vi "Close Session.vi"(8 "error in":errorcluster, 10 "Session In":T1, 11 "Text Session":refnum<class "Text Device Session.lvclass">) -> (0 "error out":errorcluster, 2 "Session Out":T1)   [LabVIEW 2018, in "Text Device Session.lvclass"]
uses:
  Text Device Session.lvclass
  <vilib>/MSR Consulting, LLC/General Reuse/Session APIs/_Session Fwk/Typedefs/Session Handle.ctl
  <vilib>/MSR Consulting, LLC/General Reuse/Session APIs/_Session Fwk/Session - Root.lvclass
  C:/Program Files (x86)/National Instruments/LabVIEW 2018/vi.lib/MSR Consulting, LLC/General Reuse/Session APIs/_Session Fwk/Session - Root.lvclass
  File Access/Config Data/Config Data.lvclass
  Session Log/System Log.lvclass
  Text Device Session.lvclass/Text Device Session.ctl
  Read hSysLog.vi
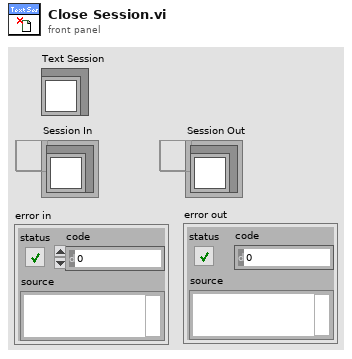
[diagram p1: front panel]
types:
  T1 = typedef "Session - Root.lvclass/Session Handle.ctl" = refnum<data-value>
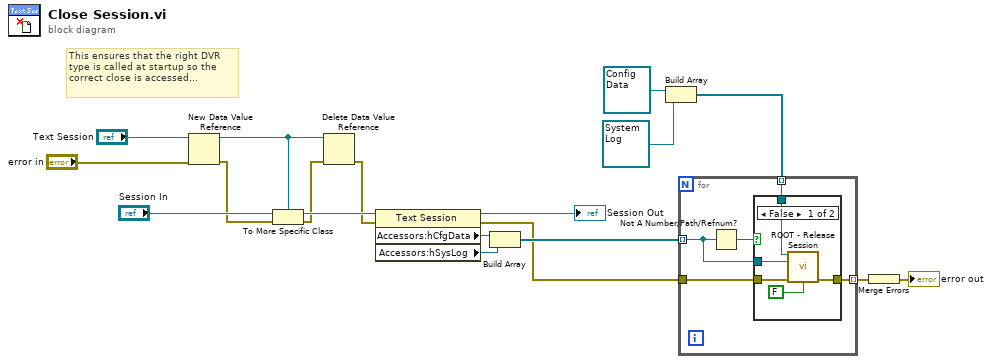
[diagram p0: block diagram]
diagram:
  # "This ensures that the right DVR type is called at startup so the correct close is accessed..."
  n1 = New Data Value Reference(data value="Text Session", error in="error in") -> (data value reference=w6:refnum<data-value>, error out=w9:errorcluster)
  n2 = To More Specific Class(target class=w6, reference="Session In", error in=w9) -> (specific class reference=w17:refnum<data-value>, error out=w8:errorcluster)
  n3 = Delete Data Value Reference(data value reference=w6, error in=w8) -> (error out=w7:errorcluster)  [unwired: 1 out]
  n4 = property class="Text Session"(reference=w17, error in=w7) -> (reference out=→"Session Out":refnum<data-value>, error out=w4:errorcluster, "Accessors:hCfgData"=w16:T1, "Accessors:hSysLog"=w15:T1)
  n5 = Build Array(w16, w15) -> (w14:T1[])
  n6 = Build Array(refnum<class "Config Data.lvclass"> refnum ("Config Data"), refnum<class "System Log.lvclass"> refnum ("Sys Log")) -> (w5:refnum<class "Session - Root.lvclass">[])
  n7 = for {
    tunnel: w14 -> [w20] mode=indexing
    tunnel: w5 -> [w23] mode=indexing
    tunnel: w4 -> [w22]
    tunnel: [w21] -> w3 mode=indexing
    n8 = Not A Number/Path/Refnum?(number/path/refnum=w20) -> (NaN/Path/Refnum?=w19:bool)
    n9 = case shown="False" w19 {
      tunnel: w23 -> [w28 _]
      tunnel: w22 -> [w26 w29]
      tunnel: [w25 w29] -> w21
      tunnel: w20 -> [w24 _]
      frame False {
        n10 = call <vilib>:"ROOT - Release Session.vi"("OBJ - Session in"=w28, "Session Handle in"=w24, "error in (no error)"=w26, "force destroy? (F)"=FALSE) -> ("error out"=w25:errorcluster)  [unwired: 10 in, 1 out]
      }
      frame True {
      }
    }
  }
  n11 = Merge Errors(w3) -> (→"error out":errorcluster)
